vi "Remove Nested Queue.vi"(8 "error in (no error)":errorcluster, 11 "Generic Actor in":refnum<class "Generic Actor.lvclass">) -> (0 "error out":errorcluster, 3 "Generic Actor out":refnum<class "Generic Actor.lvclass">)   [LabVIEW 2020, in "Generic Actor.lvlib" / "Generic Actor.lvclass"]
uses:
  Generic Actor.lvclass
  <vilib>/ActorFramework/Message Enqueuer/Message Enqueuer.lvclass
  Generic Actor.lvclass/Generic Actor.ctl
panel:
  out "Removed Nested Queue":refnum<class "Message Enqueuer.lvclass">
  out "not found?":bool
  in  "Nested Name":string
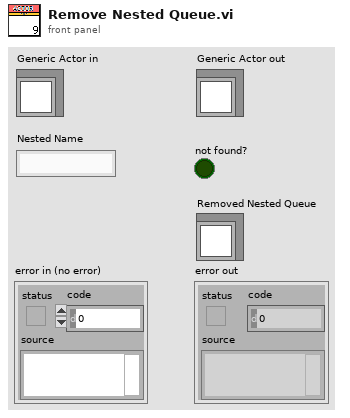
[diagram p1: front panel]
types:
  T1 = map{string, refnum<class "Message Enqueuer.lvclass">}
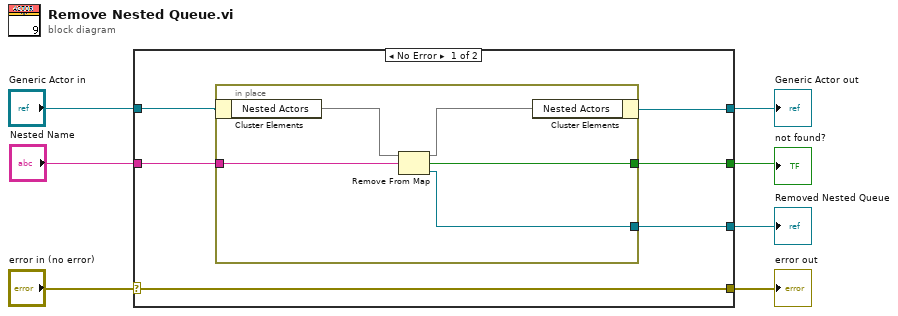
[diagram p0: block diagram]
diagram:
  n1 = case shown="No Error" "error in (no error)" {
    selector: "error in (no error)" -> [w13 w20]
    tunnel: [w13 w20] -> w6
    tunnel: [w11 w19] -> w4
    tunnel: "Generic Actor in" -> [w12 w19]
    tunnel: "Nested Name" -> [w10 _]
    tunnel: [w9 _] -> w2
    tunnel: [w8 _] -> w1
    frame No Error {
      n2 = in-place {
        in-place-border: w10 -> [w16]
        in-place-border: [w15] -> w9
        in-place-border: [w14] -> w8
        n3 = in-place-cluster #1(w12) -> ("Nested Actors"=w18:T1)
        n4 = Remove From Map(10:w16, 11:w18) -> (1:w14:refnum<class "Message Enqueuer.lvclass">, 2:w15:bool, 3:w17:T1)
        n5 = in-place-cluster #1("Nested Actors"=w17) -> (w11:refnum<class "Generic Actor.lvclass">)
      }
    }
    frame Error {
    }
  }
  "error out" <- w6
  "Generic Actor out" <- w4
  "not found?" <- w2
  "Removed Nested Queue" <- w1
